vi "Keep String in Array.vi"(9 "Current Index":i32, 10 "Max Number of Strings (8)":i32=8, 11 "Number of Elements":i32) -> (3 "Keep String":bool)   [LabVIEW 2021, in "Strings.lvlib"]
uses:
  Strings.lvlib
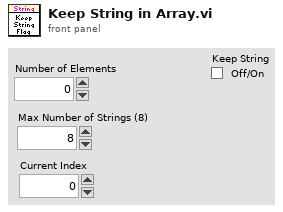
[diagram p1: front panel]
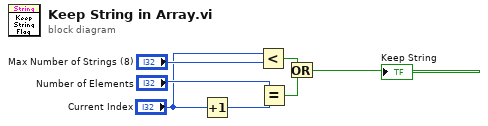
[diagram p0: block diagram]
diagram:
  n1 = Increment(x="Current Index") -> (x+1=w1:i32)
  n2 = Less?(x="Current Index", y="Max Number of Strings (8)") -> (x < y?=w6:bool)
  n3 = Equal?(x="Number of Elements", y=w1) -> (x = y?=w5:bool)
  n4 = Or(x=w6, y=w5) -> (x .or. y?=→"Keep String":bool)
